vi "DIO64 Out Status.vi"(0 "board in":u16 format="%.0x", 11 "error in (no error)":errorcluster) -> (4 "board out":u16 format="%.0x", 8 "Out Status":T1 {"startTime0" format="%.0x"; "startTime1" format="%.0x"; "cur trans" format="%.0x"; "cur reps" format="%.0x"; "#trans" format="%.0x"; "reps" format="%.0x"; "stopTime1" format="%.0x"; "stopTime0" format="%.0x"; "pktsize" format="%.0x"; "flags" format="%.0x"; "AICurrent" format="%.0x"; "startControl" format="%.0x"; "stopControl" format="%.0x"; "AIControl" format="%.0x"; "clkControl" format="%.0x"; "time0" format="%.0x"; "time1" format="%.0x"; "ticks" format="%.0x"; "readPtr" format="%.0x"; "writePtr" format="%.0x"; "fifo0" format="%.0x"; "fifoSize" format="%.0x"; "portCount" format="%.0x"}, 10 "scans available":u32, 15 "error out":errorcluster)   [LabVIEW 2012]
doc: "DIO64 Out Status checks the output status of the selected digital I/O board.\n\n\nCopyright (c) 2002 Viewpoint Systems Inc. All Rights Reserved"
uses:
  DIO64 Out Status.ctl
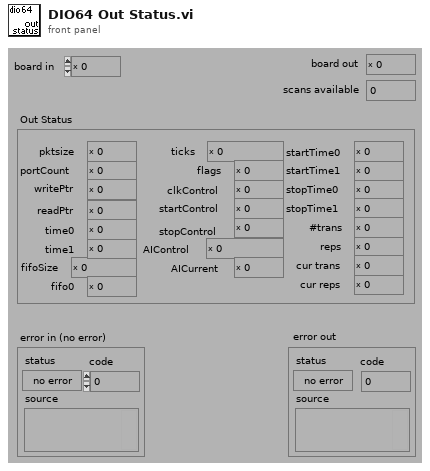
[diagram p1: front panel]
types:
  T1 = typedef "DIO64 Out Status.ctl" = cluster{"pktsize":u16, "portCount":u16, "writePtr":u16, "readPtr":u16, "time0":u16, "time1":u16, "fifoSize":u32, "fifo0":u16, "ticks":u32, "flags":u16, "clkControl":u16, "startControl":u16, "stopControl":u16, "AIControl":u32, "AICurrent":u16, "startTime0":u16, "startTime1":u16, "stopTime0":u16, "stopTime1":u16, "#trans":u16, "reps":u16, "cur trans":u16, "cur reps":u16}
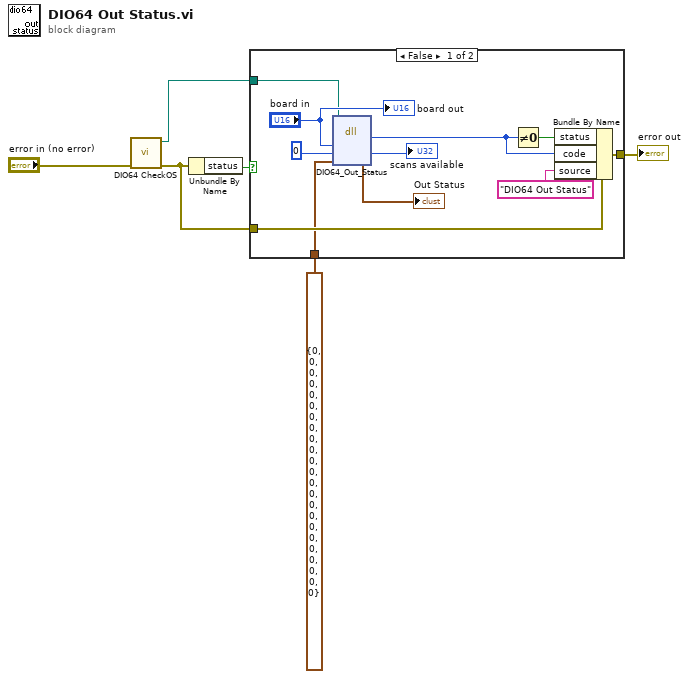
[diagram p0: block diagram]
diagram:
  n1 = call "DIO64 CheckOS.vi"("error in"="error in (no error)") -> ("error out"=w2:errorcluster, "path in"=w1:path)  [unwired: 9 in]
  n2 = Unbundle By Name(w2) -> ("status"=w6:bool)
  n3 = case shown="False" w6 {
    tunnel: w2 -> [w17 w18]
    tunnel: [w14 w18] -> w5
    tunnel: T1 {"pktsize"=0, "portCount"=0, "writePtr"=0, "readPtr"=0, "time0"=0, "time1"=0, "fifoSize"=0, "fifo0"=0, "ticks"=0, "flags"=0, "clkControl"=0, "startControl"=0, "stopControl"=0, "AIControl"=0, "AICurrent"=0, "startTime0"=0, "startTime1"=0, "stopTime0"=0, "stopTime1"=0, "#trans"=0, "reps"=0, "cur trans"=0, "cur reps"=0} ("Out Status") -> [w9 _]
    tunnel: w1 -> [w7 _]
    frame False {
      n4 = dll-call lib="C:/DIO64Visa/DLL/DIO64_Visa32/Debug/DIO64_Visa32.dll" fn="DIO64_Out_Status"(path in=w7, "board"="board in", "scansAvail"=u32 0, "status"=w9) -> ("return type"=w15:i32, "scansAvail"=→"scans available":u32, "status"=→"Out Status":T1)  [unwired: 3 in, 2 out]
      n5 = Not Equal To 0?(x=w15) -> (x != 0?=w16:bool)
      n6 = Bundle By Name(cluster=w17, "status"=w16, "code"=w15, "source"="DIO64 Out Status") -> (w14:errorcluster)
      "board out" <- "board in"
    }
    frame True {
    }
  }
  "error out" <- w5
